vi "Overview Camera.vi"(7 "Calling VI Ref":refnum<vi>) -> ()   [LabVIEW 2021]
uses:
  Overview Camera Type Defs/Overview Camera Notifier Type.ctl
  Overview Camera Type Defs/Overview Camera Actions.ctl
  <vilib>/Utility/miscctls.llb/LVPointTypeDef.ctl
  Hardware Configuration/Hardware Configuration Controls/Device Type.ctl
  Hardware Configuration/Hardware Configuration Controls/Device Function.ctl
  Device Library/Cameras/Camera Controls/Generic Camera Actions.ctl
  <vilib>/vision/Image Controls.llb/IMAQ Image.ctl
  shell32.dll
panel:
  in  "Pixel Binning":u16=1
  in  "Image Display":bool
  in  "Capture":bool
  in  "Preview":bool
  in  "Quit":bool
  out "Current Frame":u32=1
  in  "Exposure Time (s)":dbl=0.1
  in  "Base Save Path":path
  in  "File Name":string="Test Image"
  in  "Number of Frames":u32=1
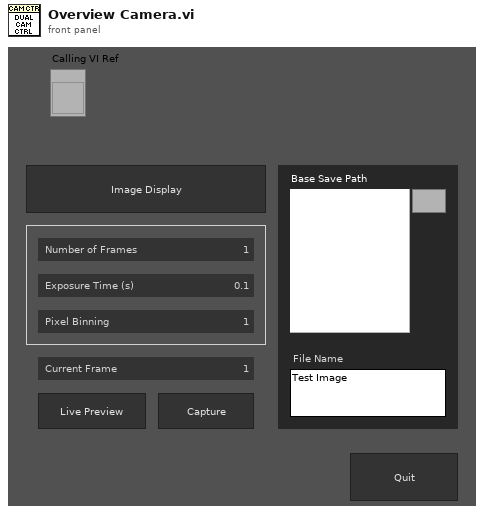
[diagram p1: front panel]
types:
  T1 = typedef "Generic Camera Actions.ctl" = enum16{"Status", "Live Preview", "Capture", "Abort", "Set Exposure Time (s)", "Get Exposure Time (s)", "Set Gain", "Get Gain", "Set Gamma", "Get Gamma", "Record Settings", "Set ROI", "Get ROI", "Binning", "Defect Correction On/Off", "Cooler On/Off", "Fan On/Off", "Quit"}
  T2 = typedef "Device Function.ctl" = enum16{"Primary", "Secondary", "Overview", "Wide Field Drift Correction", "642 nm Excitation", "560 nm Excitation", "940 nm Excitation", "546 nm Excitation", "488 nm Excitation", "405 nm Excitation", "Objective Drift Correction", "4Pi Focus Lock", "4Pi Objective Lock", "Objective XY", "Objective Z", "Sample XY", "Sample Coarse Z", "Sample Z", "4Pi Lower", "4Pi Upper", "Em Small", "Em Large", "Ex Small", "Ex Large", "Mojo", "Adj Cavity", "Line Scanning", "Alert"}
  T3 = typedef "Device Type.ctl" = enum16{"AOTF", "Camera", "Deformable Mirror", "Laser", "Flip Mirror", "Shutter", "Stage", "Waveform", "FPGA", "Filter Wheel", "Email"}
  T4 = enum16{"Always On", "Always Off", "Off While Running"}
  T5 = typedef "LVPointTypeDef.ctl" = cluster{"Horizontal":i16, "Vertical":i16}
  T6 = typedef "Overview Camera Actions.ctl" = enum16{"Idle", "Exposure Time", "Binning", "Preview", "Capture", "Set Save Path", "Start Acquisition", "Abort", "Exit Loop", "Quit"}
  T7 = typedef "Overview Camera Notifier Type.ctl" = cluster{"Actions":T6, "Exposure Time (s)":dbl, "Num of Frames":u32, "Save Path":path, "Running?":bool, "Binning":u16}
  T8 = typedef "IMAQ Image.ctl" = refnum<image>
  T9 = typedef "LVRectTypeDef.ctl" = cluster{"Left":i16, "Top":i16, "Right":i16, "Bottom":i16}
  T10 = typedef "LVBoundsTypeDef.ctl" = cluster{"Width":u32, "Height":u32}
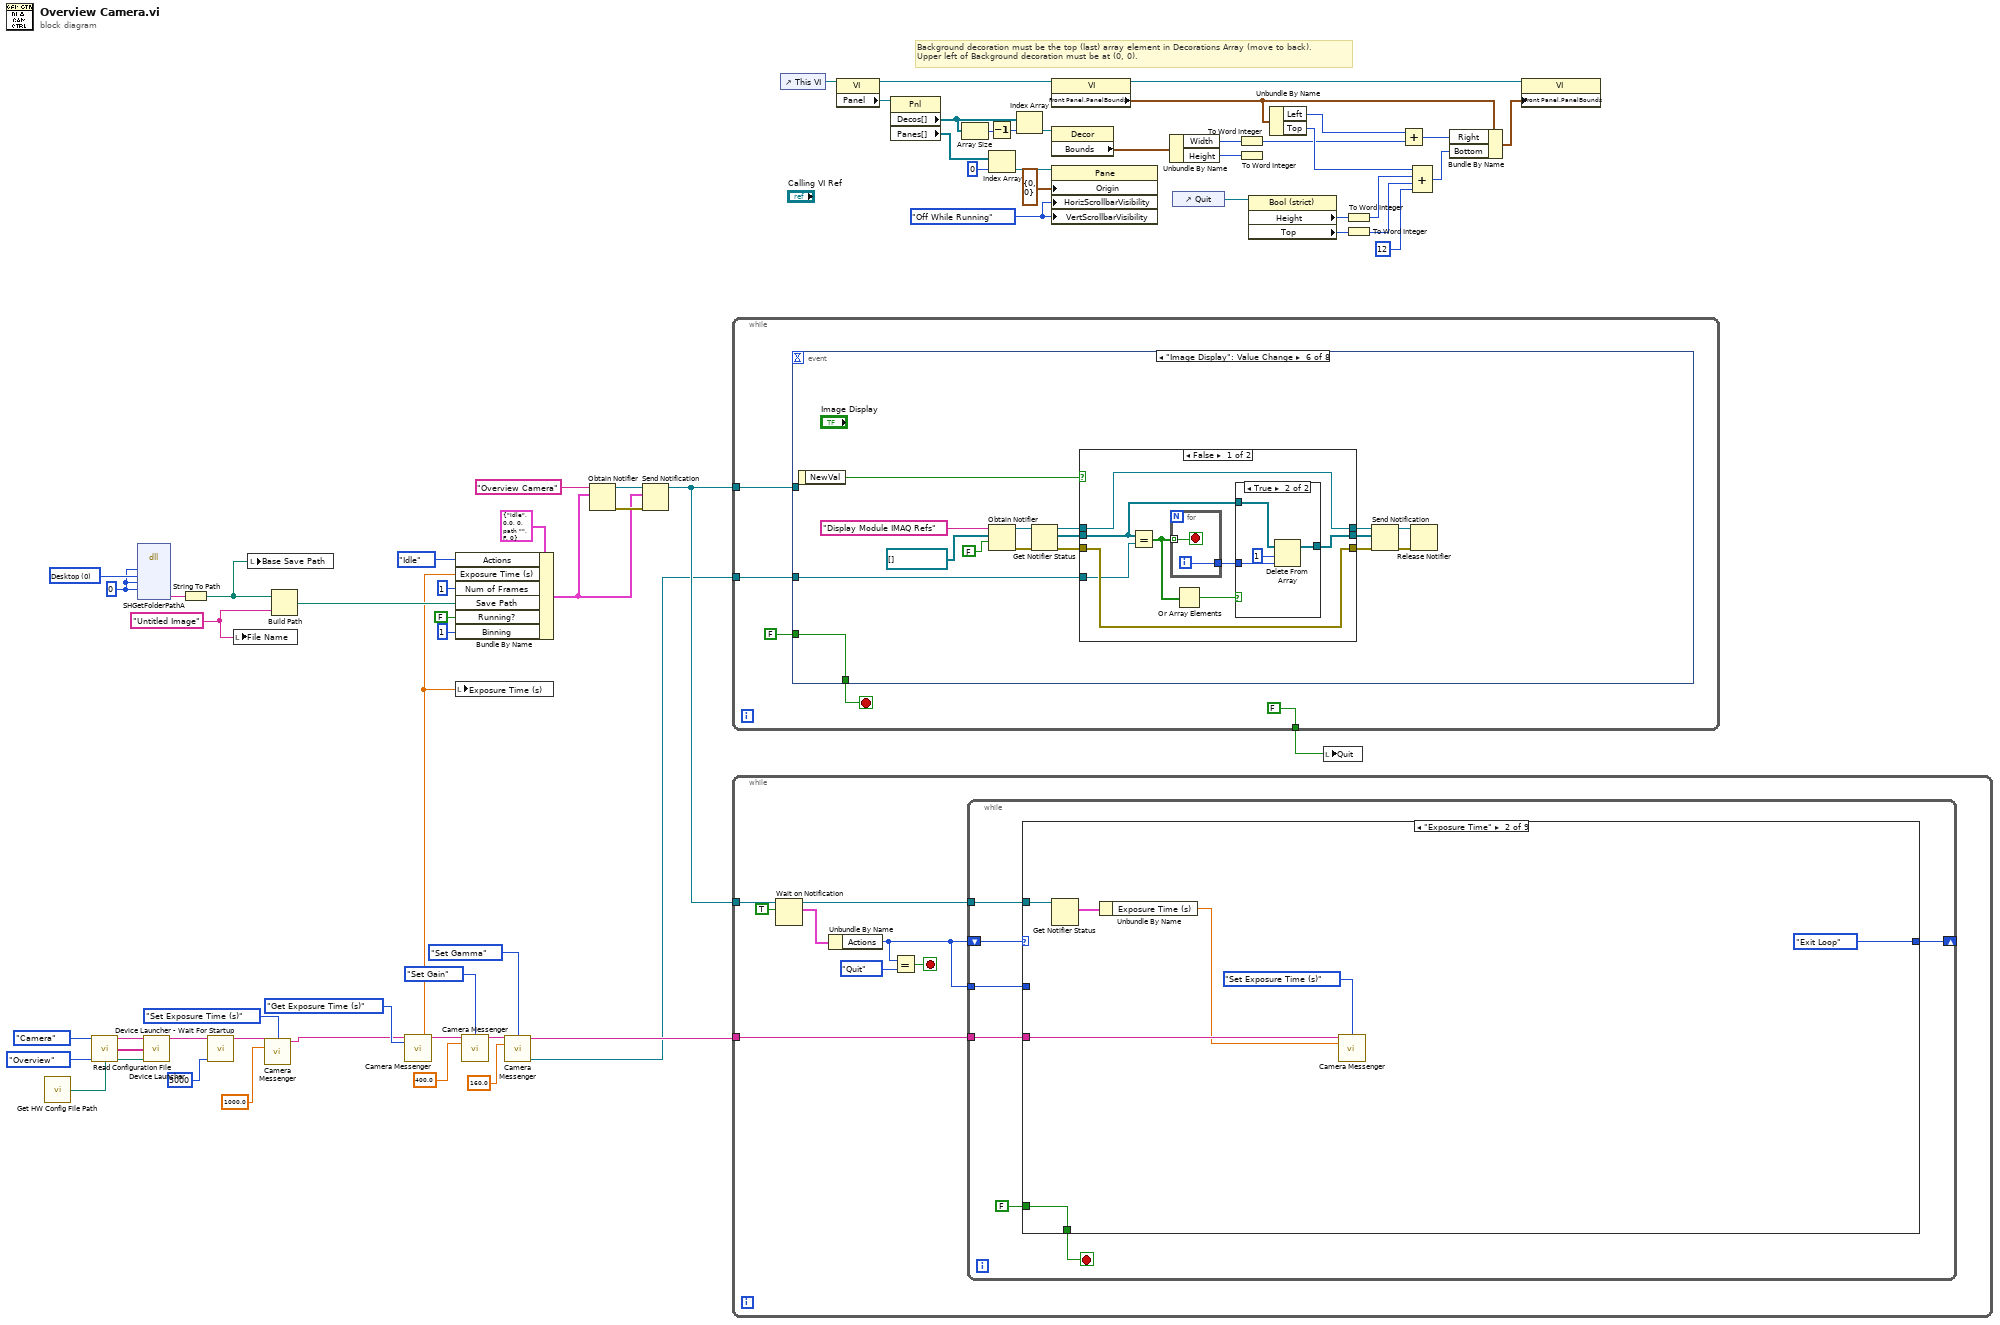
[diagram p0: block diagram]
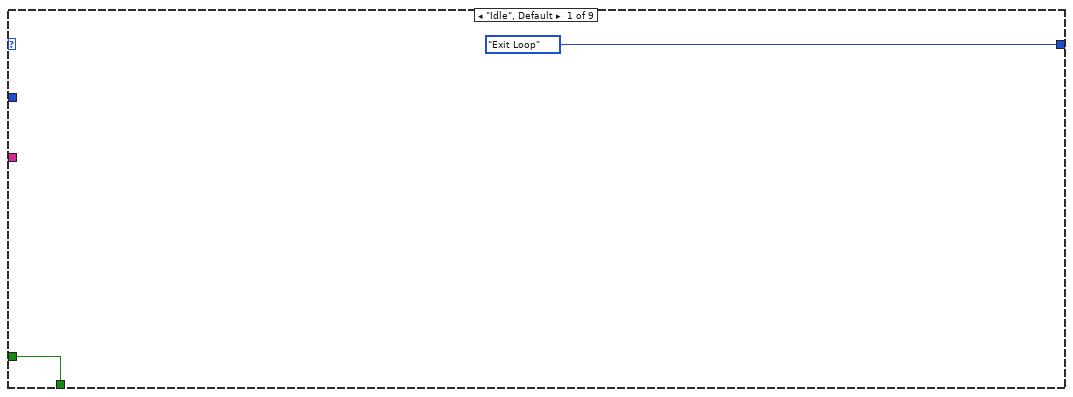
[diagram p2: hidden frame]
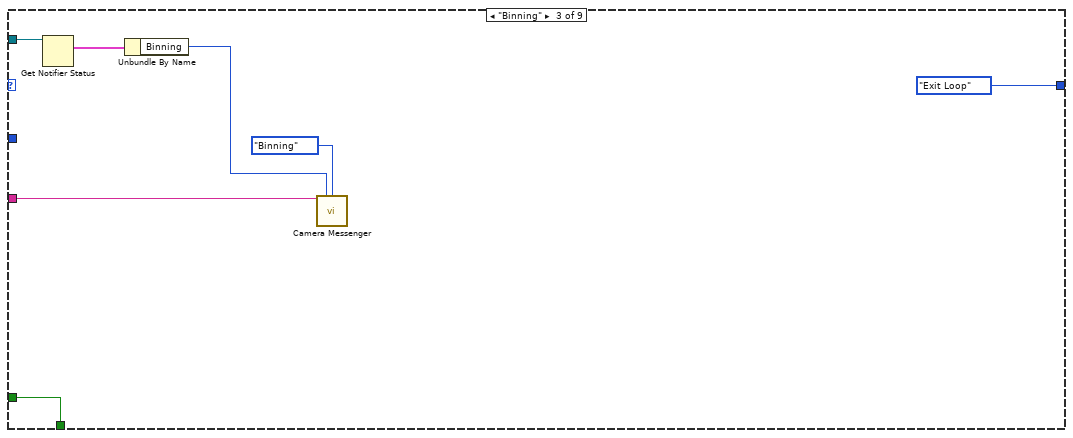
[diagram p3: hidden frame]
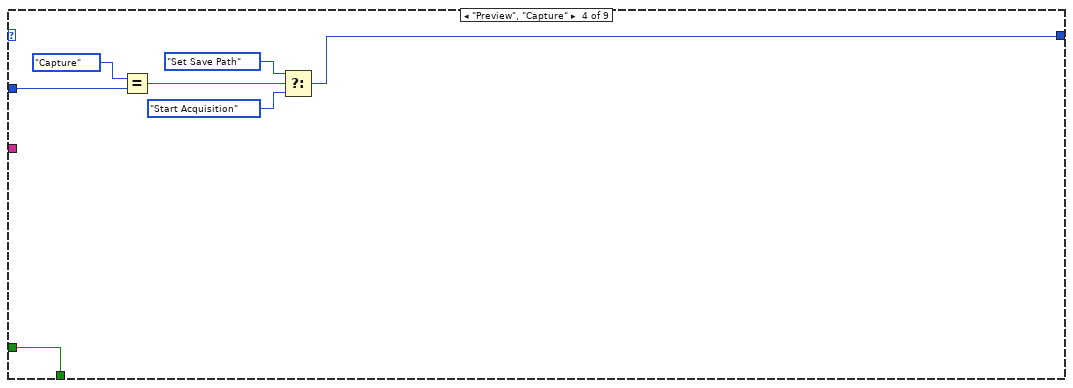
[diagram p4: hidden frame]
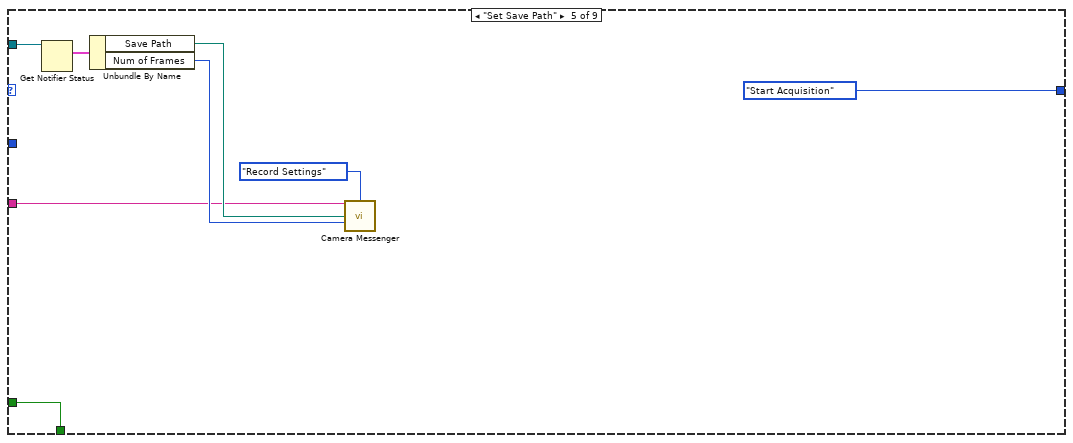
[diagram p5: hidden frame]
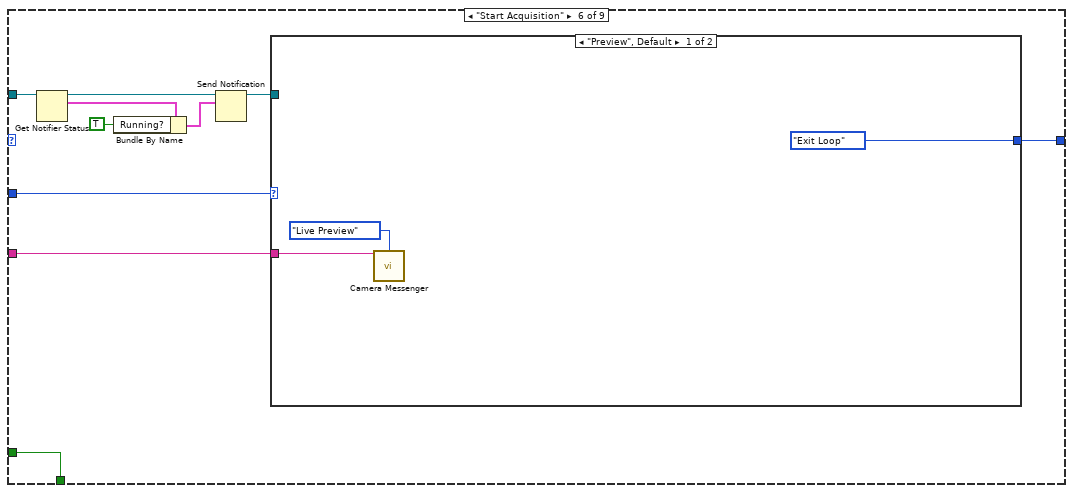
[diagram p6: hidden frame]
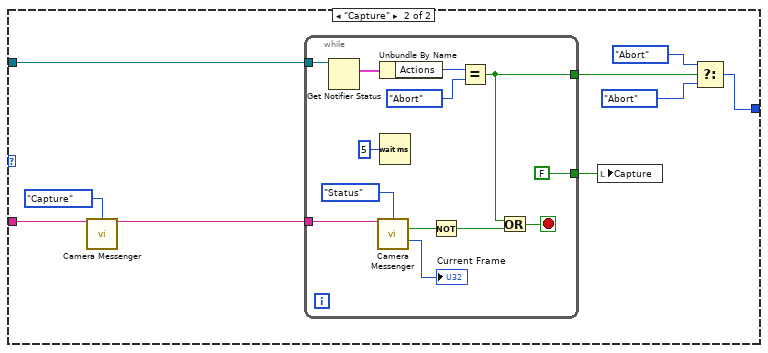
[diagram p7: hidden frame]
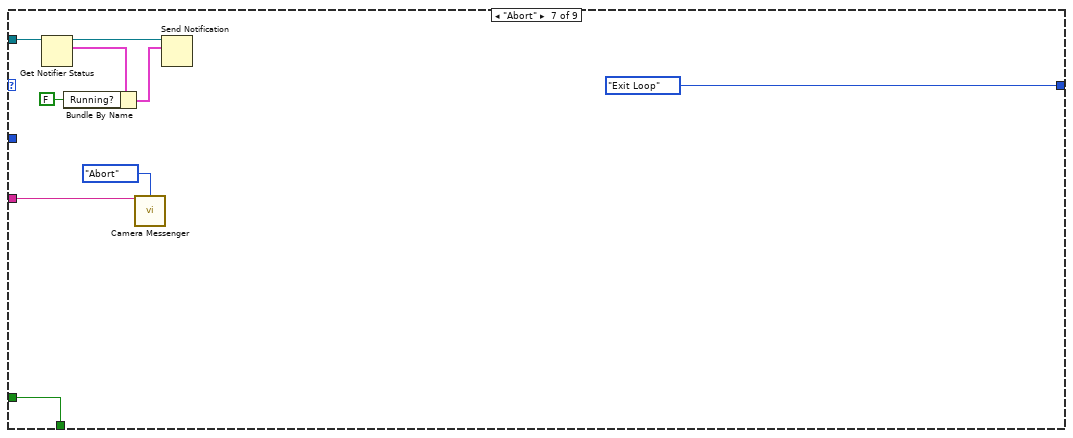
[diagram p8: hidden frame]
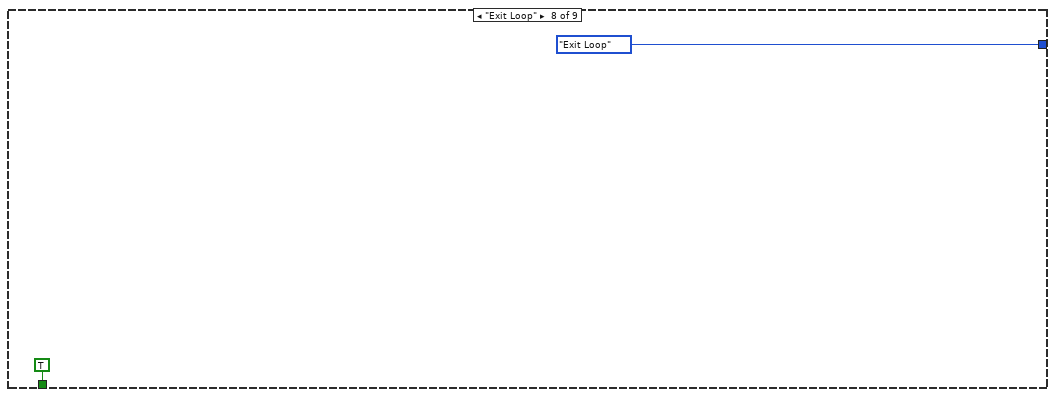
[diagram p9: hidden frame]
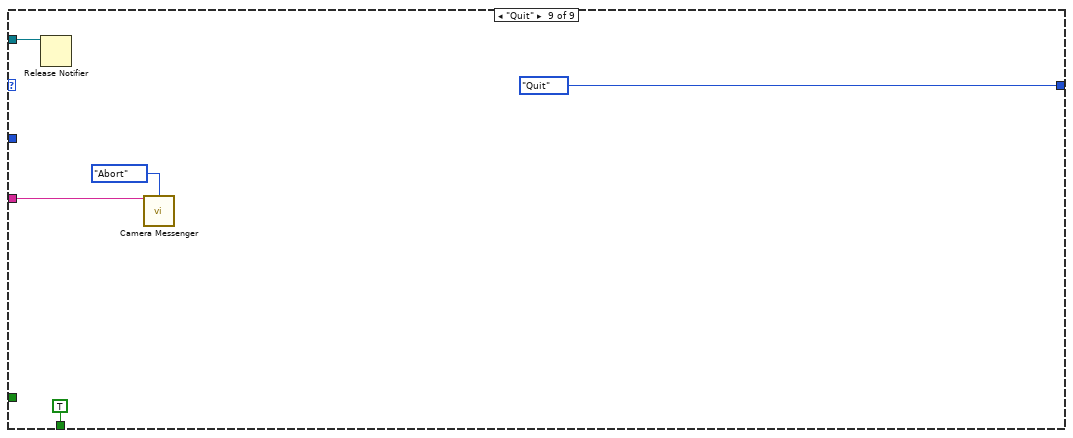
[diagram p10: hidden frame]
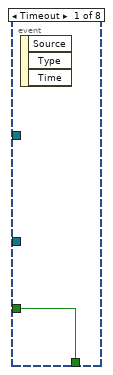
[diagram p11: hidden frame]
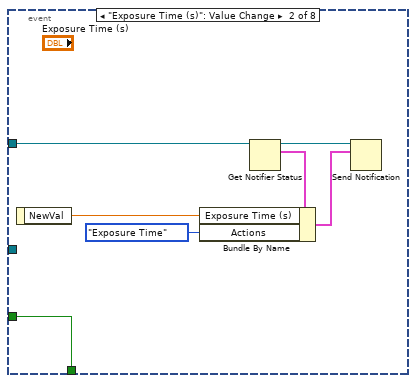
[diagram p12: hidden frame]
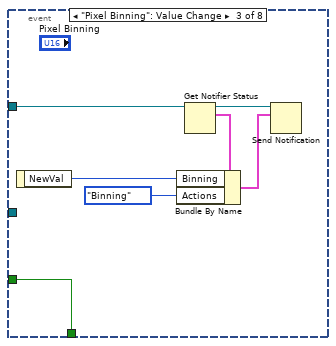
[diagram p13: hidden frame]
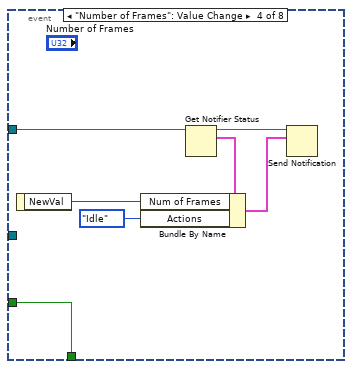
[diagram p14: hidden frame]
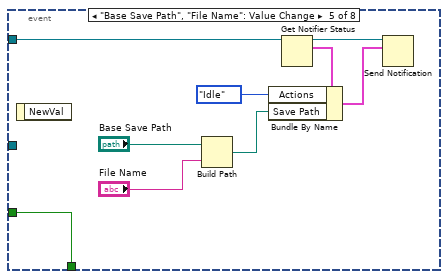
[diagram p15: hidden frame]
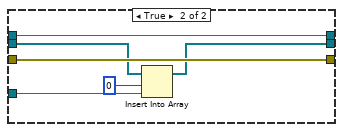
[diagram p17: hidden frame]
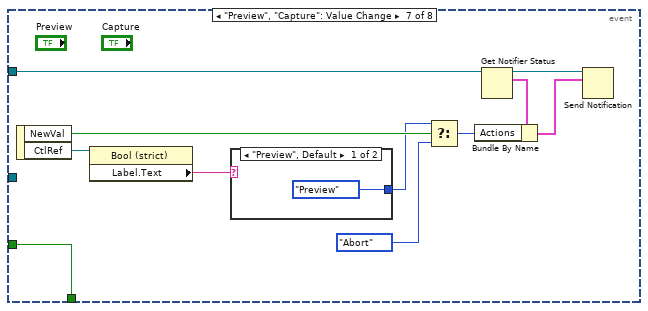
[diagram p18: hidden frame]
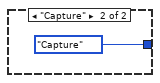
[diagram p19: hidden frame]
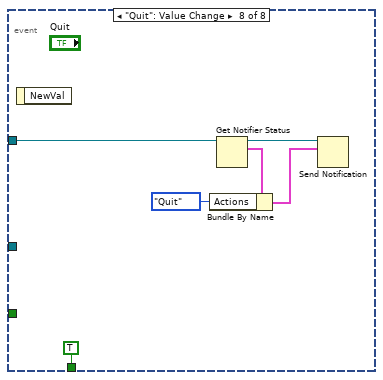
[diagram p20: hidden frame]
diagram:
  w34 = T4."Off While Running" ("Vertical Scrollbar Visibility")
  w64 = "Untitled Image"
  w67 = 0 items=["Desktop"=0, "Personal Documents"=5, "AppData"=26, "Local AppData"=28, "Common AppData"=35, "Program Files"=38, "Program Files Common"=43, "Common Documents"=46] ("Requested Path")
  w66 = 0 ("HWND")
  # "Background decoration must be the top (last) array element in Decorations Array (move to back).\nUpper left of Background decoration must be at (0, 0)."
  n1 = call "Get HW Config File Path.vi"() -> ("File Path"=w52:path)  [unwired: 14 in, 1 out]
  n2 = call "Read Configuration File.vi"("Device Type"=Device_Type."Camera", "Device Function"=Device_Function."Overview", "Config File Path"=w52) -> ("Unique Notifier Name"=w20:string, "Device Ports/IDs/Channels"=w22:string[], "Device Engine Path"=w21:path)  [unwired: 9 in, 1 out]
  n3 = dll-call lib="shell32.dll" fn="SHGetFolderPathA"("HWND"=w66, "nFolder"=w67, "hToken"=w66, "dwFlags"=w66) -> ("pszPath"=w65:string)  [unwired: 9 in, 2 out]
  n4 = call "Device Launcher.vi"("Notifier Name"=w20, "Device Ports/IDs/Channels"=w22, "Device Engine Path"=w21) -> ("Notifier Name"=w18:string)  [unwired: 11 in, 1 out]
  n5 = String To Path(string=w65) -> (path=w63:path)
  n6 = call "Device Launcher - Wait For Startup.vi"("Notifier Name"=w18, "Wait Time (ms)"=5000) -> ("Notifier Name (Dup)"=w4:string)  [unwired: 12 in, 1 out]
  n7 = local write "File Name"(w64) -> ()
  n8 = local write "Base Save Path"(w63) -> ()
  n9 = call "Camera Messenger.vi"("Notifier Name"=w4, "General Camera Actions"=Generic_Camera_Actions."Set Exposure Time (s)", "Exposure Time (s)"=1000.0) -> ("Notifier Name Dup"=w1:string)  [unwired: 7 in, 5 out]
  n10 = Build Path(base path=w63, name or relative path=w64) -> (appended path=w59:path)
  n11 = call "Camera Messenger.vi"("Notifier Name"=w1, "General Camera Actions"=Generic_Camera_Actions."Get Exposure Time (s)") -> ("Current Exposure Time (s)"=w14:dbl, "Notifier Name Dup"=w12:string)  [unwired: 8 in, 4 out]
  n12 = Bundle By Name(cluster=T7 {"Actions"=enum."Idle", "Exposure Time (s)"=0.0, "Num of Frames"=0, "Save Path"=path "", "Running?"=FALSE, "Binning"=0} ("Dual Camera Notifier Type"), "Actions"=Overview_Camera_Actions."Idle", "Exposure Time (s)"=w14, "Num of Frames"=u32 1, "Save Path"=w59, "Running?"=FALSE, "Binning"=1) -> (w55:T7)
  n13 = local write "Exposure Time (s)"(w14) -> ()
  n14 = call "Camera Messenger.vi"("Notifier Name"=w12, "General Camera Actions"=Generic_Camera_Actions."Set Gain", "Exposure Time (s)"=400.0) -> ("Notifier Name Dup"=w9:string)  [unwired: 7 in, 5 out]
  n15 = call "Camera Messenger.vi"("Notifier Name"=w9, "General Camera Actions"=Generic_Camera_Actions."Set Gamma", "Exposure Time (s)"=160.0) -> ("Notifier Name Dup"=w6:string, "Image Ref"=w5:T8)  [unwired: 7 in, 4 out]
  n16 = Obtain Notifier(name (unnamed)="Overview Camera", notification data type=w55) -> (notifier out=w57:refnum<notifier>, error out=w56:errorcluster)  [unwired: 2 in, 1 out]
  n17 = Send Notification(notification=w55, notifier=w57, error in (no error)=w56) -> (notifier out=w53:refnum<notifier>)  [unwired: 1 out]
  n18 = while {
    tunnel: w53 -> [w71]
    tunnel: [FALSE] -> w54
    tunnel: w5 -> [w69]
    stop <- w72 stop-if-true
    n19 = event shown="[5] \"Image Display\": Value Change" {
      selector: _ -> [_ _ _ _ _ _ _ _]
      dyn-events: _ -> [_ _ _ _ _ _ _ _]
      timeout: _ -> [_ _ _ _ _ _ _ _]
      tunnel: FALSE -> [w74 w81 w88 w95 w104 w120 w152 _]
      tunnel: [w74 w81 w88 w95 w104 w120 w152 TRUE] -> w72
      tunnel: w71 -> [_ w80 w83 w94 w103 _ w151 w156]
      tunnel: w69 -> [_ _ _ _ _ w105 _ _]
      event Timeout {
        n20 = event-data() -> ()  [unwired: 1 in, 3 out]
      }
      event "Exposure Time (s)": Value Change {
        n21 = event-data() -> ("NewVal"=w78:dbl)  [unwired: 1 in]
        n22 = Get Notifier Status(notifier=w80) -> (notifier out=w76:refnum<notifier>, current notification=w79:T7)  [unwired: 1 in, 3 out]
        n23 = Bundle By Name(cluster=w79, "Exposure Time (s)"=w78, "Actions"=Overview_Camera_Actions."Exposure Time") -> (w75:T7)
        n24 = Send Notification(notification=w75, notifier=w76) -> ()  [unwired: 1 in, 2 out]
      }
      event "Pixel Binning": Value Change {
        n25 = event-data() -> ("NewVal"=w82:u16)  [unwired: 1 in]
        n26 = Get Notifier Status(notifier=w83) -> (notifier out=w85:refnum<notifier>, current notification=w87:T7)  [unwired: 1 in, 3 out]
        n27 = Bundle By Name(cluster=w87, "Binning"=w82, "Actions"=Overview_Camera_Actions."Binning") -> (w84:T7)
        n28 = Send Notification(notification=w84, notifier=w85) -> ()  [unwired: 1 in, 2 out]
      }
      event "Number of Frames": Value Change {
        n29 = event-data() -> ("NewVal"=w92:u32)  [unwired: 1 in]
        n30 = Get Notifier Status(notifier=w94) -> (notifier out=w90:refnum<notifier>, current notification=w93:T7)  [unwired: 1 in, 3 out]
        n31 = Bundle By Name(cluster=w93, "Num of Frames"=w92, "Actions"=Overview_Camera_Actions."Idle") -> (w89:T7)
        n32 = Send Notification(notification=w89, notifier=w90) -> ()  [unwired: 1 in, 2 out]
      }
      event "Base Save Path", "File Name": Value Change {
        n33 = event-data() -> ()  [unwired: 1 in, 1 out]
        n34 = Build Path(base path="Base Save Path", name or relative path="File Name") -> (appended path=w96:path)
        n35 = Get Notifier Status(notifier=w103) -> (notifier out=w101:refnum<notifier>, current notification=w102:T7)  [unwired: 1 in, 3 out]
        n36 = Bundle By Name(cluster=w102, "Actions"=Overview_Camera_Actions."Idle", "Save Path"=w96) -> (w100:T7)
        n37 = Send Notification(notification=w100, notifier=w101) -> ()  [unwired: 1 in, 2 out]
      }
      event "Image Display": Value Change {
        n38 = event-data() -> ("NewVal"=w106:bool)  [unwired: 1 in]
        n39 = Obtain Notifier(name (unnamed)="Display Module IMAQ Refs", notification data type=T8[] [], create if not found? (T)=FALSE) -> (notifier out=w113:refnum<notifier>, error out=w112:errorcluster)  [unwired: 1 in, 1 out]
        n40 = Get Notifier Status(notifier=w113, error in (no error)=w112) -> (notifier out=w114:refnum<notifier>, current notification=w116:T8[], error out=w115:errorcluster)  [unwired: 2 out]
        n41 = case shown="False" w106 {
          tunnel: w114 -> [w128 w141]
          tunnel: w115 -> [w122 w140]
          tunnel: w116 -> [w124 w139]
          tunnel: [w123 w136] -> w119
          tunnel: [w128 w141] -> w117
          tunnel: [w122 w140] -> w118
          tunnel: w105 -> [w121 w138]
          frame False {
            n42 = Equal?(x=w124, y=w121) -> (x = y?=w127:bool[])
            n43 = for {
              tunnel: w127 -> [w135] mode=indexing
              tunnel: [w134] -> w125
              i -> [w134]
              stop <- w135 stop-if-true
            }
            n44 = Or Array Elements(Boolean array=w127) -> (logical OR=w126:bool)
            n45 = case shown="True" w126 {
              tunnel: w125 -> [_ w132]
              tunnel: w124 -> [w129 w131]
              tunnel: [w129 w130] -> w123
              frame False {
              }
              frame True {
                n46 = Delete From Array(array=w131, length=1, index=w132) -> (array with subset deleted=w130:T8[])  [unwired: 1 out]
              }
            }
          }
          frame True {
            n47 = Insert Into Array(array=w139, index=0, new element=w138) -> (w136:T8[])
          }
        }
        n48 = Send Notification(notification=w119, notifier=w117, error in (no error)=w118) -> (notifier out=w111:refnum<notifier>, error out=w110:errorcluster)
        n49 = Release Notifier(notifier=w111, error in (no error)=w110) -> ()  [unwired: 1 in, 3 out]
      }
      event "Preview", "Capture": Value Change {
        n50 = event-data() -> ("NewVal"=w146:bool, "CtlRef"=w147:refnum<vi>)  [unwired: 1 in]
        n51 = property class="Bool (strict)"(reference=w147) -> ("Label.Text"=w144:string)  [unwired: 1 in, 2 out]
        n52 = case shown="\"Preview\", Default" w144 {
          tunnel: [Overview_Camera_Actions."Preview" ("Actions") Overview_Camera_Actions."Capture" ("Actions")] -> w143
          frame "Preview", Default {
          }
          frame "Capture" {
          }
        }
        n53 = Select(t=w143, s=w146, f=Overview_Camera_Actions."Abort" ("Actions")) -> (s? t:f=w145:T6)
        n54 = Get Notifier Status(notifier=w151) -> (notifier out=w149:refnum<notifier>, current notification=w150:T7)  [unwired: 1 in, 3 out]
        n55 = Bundle By Name(cluster=w150, "Actions"=w145) -> (w148:T7)
        n56 = Send Notification(notification=w148, notifier=w149) -> ()  [unwired: 1 in, 2 out]
      }
      event "Quit": Value Change {
        n57 = event-data() -> ()  [unwired: 1 in, 1 out]
        n58 = Get Notifier Status(notifier=w156) -> (notifier out=w158:refnum<notifier>, current notification=w157:T7)  [unwired: 1 in, 3 out]
        n59 = Bundle By Name(cluster=w157, "Actions"=Overview_Camera_Actions."Quit") -> (w159:T7)
        n60 = Send Notification(notification=w159, notifier=w158) -> ()  [unwired: 1 in, 2 out]
      }
    }
  }
  n61 = while {
    tunnel: w53 -> [w168]
    tunnel: w6 -> [w162]
    stop <- w164 stop-if-true
    n62 = Wait on Notification(notifier=w168, ignore previous (F)=TRUE) -> (notifier out=w163:refnum<notifier>, notification=w166:T7)  [unwired: 2 in, 2 out]
    n63 = Unbundle By Name(w166) -> ("Actions"=w161:T6)
    n64 = Equal?(x=w161, y=Overview_Camera_Actions."Quit" ("Actions")) -> (x = y?=w164:bool)
    n65 = while {
      shift-right: [w170] -> _
      shift-left: w161 -> [w174]
      tunnel: w163 -> [w175]
      tunnel: w162 -> [w171]
      tunnel: w161 -> [w169]
      stop <- w172 stop-if-true
      n66 = case shown="\"Exposure Time\"" w174 {
        tunnel: w175 -> [_ w182 w189 _ w204 w214 w247 _ w257]
        tunnel: FALSE -> [w177 w183 w190 w198 w206 w216 w250 _ _]
        tunnel: [w177 w183 w190 w198 w206 w216 w250 TRUE TRUE] -> w172
        tunnel: w171 -> [_ w181 w188 _ w199 w207 w249 _ w256]
        tunnel: [Overview_Camera_Actions."Exit Loop" ("Actions") Overview_Camera_Actions."Exit Loop" ("Actions") Overview_Camera_Actions."Exit Loop" ("Actions") w196 Overview_Camera_Actions."Start Acquisition" ("Actions") w213 Overview_Camera_Actions."Exit Loop" ("Actions") Overview_Camera_Actions."Exit Loop" ("Actions") Overview_Camera_Actions."Quit" ("Actions")] -> w170
        tunnel: w169 -> [_ _ _ w197 _ w215 _ _ _]
        frame "Idle", Default {
        }
        frame "Exposure Time" {
          n67 = Get Notifier Status(notifier=w182) -> (current notification=w180:T7)  [unwired: 1 in, 4 out]
          n68 = Unbundle By Name(w180) -> ("Exposure Time (s)"=w179:dbl)
          n69 = call "Camera Messenger.vi"("Notifier Name"=w181, "General Camera Actions"=Generic_Camera_Actions."Set Exposure Time (s)", "Exposure Time (s)"=w179) -> ()  [unwired: 7 in, 6 out]
        }
        frame "Binning" {
          n70 = Get Notifier Status(notifier=w189) -> (current notification=w187:T7)  [unwired: 1 in, 4 out]
          n71 = Unbundle By Name(w187) -> ("Binning"=w185:u16)
          n72 = call "Camera Messenger.vi"("Notifier Name"=w188, "Binning"=w185, "General Camera Actions"=Generic_Camera_Actions."Binning") -> ()  [unwired: 7 in, 6 out]
        }
        frame "Preview", "Capture" {
          n73 = Equal?(x=Overview_Camera_Actions."Capture", y=w197) -> (x = y?=w193:bool)
          n74 = Select(t=Overview_Camera_Actions."Set Save Path" ("Actions"), s=w193, f=Overview_Camera_Actions."Start Acquisition" ("Actions")) -> (s? t:f=w196:T6)
        }
        frame "Set Save Path" {
          n75 = Get Notifier Status(notifier=w204) -> (current notification=w203:T7)  [unwired: 1 in, 4 out]
          n76 = Unbundle By Name(w203) -> ("Save Path"=w200:path, "Num of Frames"=w202:u32)
          n77 = call "Camera Messenger.vi"("Notifier Name"=w199, "General Camera Actions"=Generic_Camera_Actions."Record Settings", "Save Path"=w200, "No. of Frames"=w202) -> ()  [unwired: 6 in, 6 out]
        }
        frame "Start Acquisition" {
          n78 = Get Notifier Status(notifier=w214) -> (notifier out=w209:refnum<notifier>, current notification=w208:T7)  [unwired: 1 in, 3 out]
          n79 = Bundle By Name(cluster=w208, "Running?"=TRUE) -> (w211:T7)
          n80 = Send Notification(notification=w211, notifier=w209) -> (notifier out=w210:refnum<notifier>)  [unwired: 1 in, 1 out]
          n81 = case shown="\"Preview\", Default" w215 {
            tunnel: w207 -> [w219 w228]
            tunnel: w210 -> [_ w226]
            tunnel: [Overview_Camera_Actions."Exit Loop" ("Actions") w220] -> w213
            frame "Preview", Default {
              n82 = call "Camera Messenger.vi"("Notifier Name"=w219, "General Camera Actions"=Generic_Camera_Actions."Live Preview") -> ()  [unwired: 8 in, 6 out]
            }
            frame "Capture" {
              n83 = call "Camera Messenger.vi"("Notifier Name"=w228, "General Camera Actions"=Generic_Camera_Actions."Capture") -> ("Notifier Name Dup"=w225:string)  [unwired: 8 in, 5 out]
              n84 = while {
                tunnel: w226 -> [w241]
                tunnel: w225 -> [w237]
                tunnel: [FALSE] -> w224
                tunnel: [w229] -> w223
                stop <- w233 stop-if-true
                n85 = Get Notifier Status(notifier=w241) -> (current notification=w240:T7)  [unwired: 1 in, 4 out]
                n86 = call "Camera Messenger.vi"("Notifier Name"=w237, "General Camera Actions"=Generic_Camera_Actions."Status") -> ("Running?"=w235:bool, "Current Frame"=→"Current Frame":u32)  [unwired: 8 in, 4 out]
                n87 = Unbundle By Name(w240) -> ("Actions"=w239:T6)
                n88 = Wait (ms)(milliseconds to wait=u32 5) -> ()  [unwired: 1 out]
                n89 = Not(x=w235) -> (.not. x?=w234:bool)
                n90 = Equal?(x=w239, y=Overview_Camera_Actions."Abort") -> (x = y?=w229:bool)
                n91 = Or(x=w229, y=w234) -> (x .or. y?=w233:bool)
              }
              n92 = local write "Capture"(w224) -> ()
              n93 = Select(t=Overview_Camera_Actions."Abort" ("Actions"), s=w223, f=Overview_Camera_Actions."Abort" ("Actions")) -> (s? t:f=w220:T6)
            }
          }
        }
        frame "Abort" {
          n94 = Get Notifier Status(notifier=w247) -> (notifier out=w243:refnum<notifier>, current notification=w246:T7)  [unwired: 1 in, 3 out]
          n95 = Bundle By Name(cluster=w246, "Running?"=FALSE) -> (w244:T7)
          n96 = call "Camera Messenger.vi"("Notifier Name"=w249, "General Camera Actions"=Generic_Camera_Actions."Abort") -> ()  [unwired: 8 in, 6 out]
          n97 = Send Notification(notification=w244, notifier=w243) -> ()  [unwired: 1 in, 2 out]
        }
        frame "Exit Loop" {
        }
        frame "Quit" {
          n98 = Release Notifier(notifier=w257) -> ()  [unwired: 2 in, 3 out]
          n99 = call "Camera Messenger.vi"("Notifier Name"=w256, "General Camera Actions"=Generic_Camera_Actions."Abort") -> ()  [unwired: 8 in, 6 out]
        }
      }
    }
  }
  n100 = control-ref of="This VI"() -> (w26:refnum<vi>)
  n101 = property class="VI"(reference=w26) -> (reference out=w35:refnum<vi>, "Panel"=w27:refnum<vi>)  [unwired: 1 in, 1 out]
  n102 = property class="Pnl"(reference=w27) -> ("Decos[]"=w25:refnum<vi>[], "Panes[]"=w31:refnum<vi>[])  [unwired: 1 in, 2 out]
  n103 = Array Size(array=w25) -> (size(s)=w23:i32)
  n104 = Decrement(x=w23) -> (x-1=w24:i32)
  n105 = Index Array(array=w31, index=0) -> (element=w30:refnum<vi>)
  n106 = Index Array(array=w25, index=w24) -> (element=w33:refnum<vi>)
  n107 = property class="VI"(reference=w35) -> (reference out=w37:refnum<vi>, "Front Panel.PanelBounds"=w38:T9)  [unwired: 1 in, 1 out]
  n108 = property class="Decor"(reference=w33) -> ("Bounds"=w36:T10)  [unwired: 1 in, 2 out]
  n109 = property class="Pane"(reference=w30, "Origin"=T5 {"Horizontal"=0, "Vertical"=0}, "HorizScrollbarVisibility"=w34, "VertScrollbarVisibility"=w34) -> ()  [unwired: 1 in, 2 out]
  n110 = Unbundle By Name(w36) -> ("Width"=w41:u32, "Height"=w44:u32)
  n111 = control-ref of="Quit"() -> (w28:refnum<vi>)
  n112 = To Word Integer(number=w41) -> (16bit integer=w43:i16)
  n113 = To Word Integer(number=w44) -> ()  [unwired: 1 out]
  n114 = property class="Bool (strict)"(reference=w28) -> ("Height"=w46:u32, "Top"=w47:i32)  [unwired: 1 in, 2 out]
  n115 = Unbundle By Name(w38) -> ("Left"=w40:i16, "Top"=w51:i16)
  n116 = local write "Quit"(w54) -> ()
  n117 = To Word Integer(number=w46) -> (16bit integer=w49:i16)
  n118 = To Word Integer(number=w47) -> (16bit integer=w50:i16)
  n119 = Add(x=w40, y=w43) -> (x+y=w42:i16)
  n120 = Compound Arithmetic op=ADD(w51, w49, w50, i16 12 ("y")) -> (w45:i16)
  n121 = Bundle By Name(cluster=w38, "Right"=w42, "Bottom"=w45) -> (w39:T9)
  n122 = property class="VI"(reference=w37, "Front Panel.PanelBounds"=w39) -> ()  [unwired: 1 in, 2 out]
